vi "Get Slot Number.vi"(7 "error in (no error)":errorcluster, 10 "SLSC Device":refnum<k21>) -> (0 "error out":errorcluster, 3 "slot number":u32)   [LabVIEW 2017, in "NI-SWITCH Examples.lvlib"]
uses:
  NI-SWITCH Examples.lvlib
  <vilib>/SLSC/Initialize Session with Devices.vi
  <vilib>/SLSC/Close Session.vi
  <resource>/objmgr/slsc.rc
  <vilib>/SLSC/SLSC.lvlib
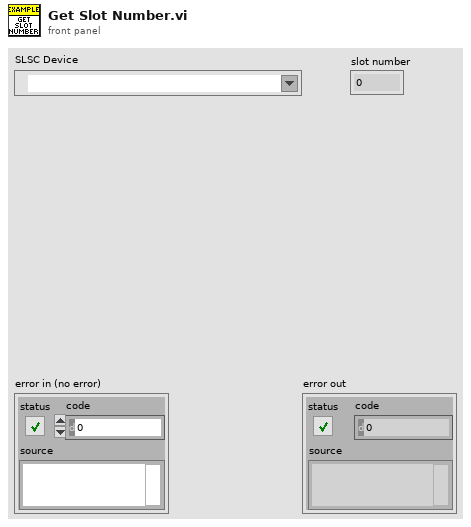
[diagram p1: front panel]
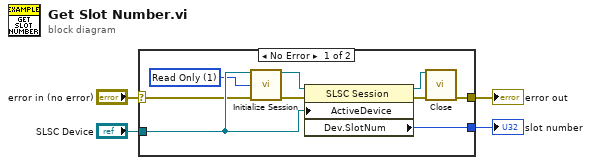
[diagram p0: block diagram]
diagram:
  n1 = case shown="No Error" "error in (no error)" {
    selector: "error in (no error)" -> [w10 w14]
    tunnel: "SLSC Device" -> [w11 _]
    tunnel: [w9 _] -> w2
    tunnel: [w5 w14] -> w1
    frame No Error {
      w6 = 1 items=["None"=0, "Read Only"=1, "Read/Write"=3] ("reservation access (Read/Write)")
      n2 = call-poly <vilib>:"Initialize Session.vi"("devices"=w11, "reservation access (Read/Write)"=w6, "error in (no error)"=w10) -> ("session out"=w13:refnum<k21>, "error out"=w12:errorcluster)  [unwired: 11 in]
      n3 = property class="SLSC Session"(reference=w13, error in=w12, "ActiveDevice"=w11) -> (reference out=w7:refnum<k21>, error out=w8:errorcluster, "Dev.SlotNum"=w9:u32)
      n4 = call-poly <vilib>:"Close.vi"("session in"=w7, "error in (no error)"=w8) -> ("error out"=w5:errorcluster)  [unwired: 13 in]
    }
    frame Error {
    }
  }
  "slot number" <- w2
  "error out" <- w1
